vi "GetErrors3.vi"(0 "XRef":T6, 1 "Generate Strings?":T1, 2 "State In":T5) -> (14 "Errors":T2, 15 "Errors Present?":T1)   [LabVIEW 2018, in "OpenG Remove Duplicates from 1 D Array.xnode"]
doc: "This ability VI is used to tell LabVIEW about errors involving your XNode instance. The Errors array is a cluster of errors that will show up as block diagram errors in LabVIEW's error window. The cluster is made up of the errors in the list, the long descriptions of the errors that show up in LabVIEW's error window's details box, and a help file and topic within that file that links this error to the specified help file via the Help button. The help file is the name of the file (*.chm), not the full path and needs to be part of LabVIEW. You only need to populate the array when Generate Strings? is true. You always need to correctly set the Errors Present? indicator. If you are generating strings, then Errors Present? should be true if and only if Errors is not empty. If errors are present, the VI containing the XNode will be broken.\n \n Remeber to localize your errors.\n\nDefault behavior: Generate generic error messages if the code you script is invalid, or a required terminal is unwired.\n\nThis ability does not provide UI and OS messages are not handled."
uses:
  OpenG Remove Duplicates from 1 D Array.xnode
  <vilib>/XNodeSupport/XNodeXNodeRef.ctl
  <vilib>/XNodeSupport/XNodeBool.ctl
  State.ctl
  <vilib>/XNodeSupport/XNodeError3Array.ctl
  <vilib>/XNodeSupport/XNodeError3.ctl
  <vilib>/XNodeSupport/XNodeString.ctl
  <vilib>/XNodeSupport/NI_XNodeSupport.lvlib
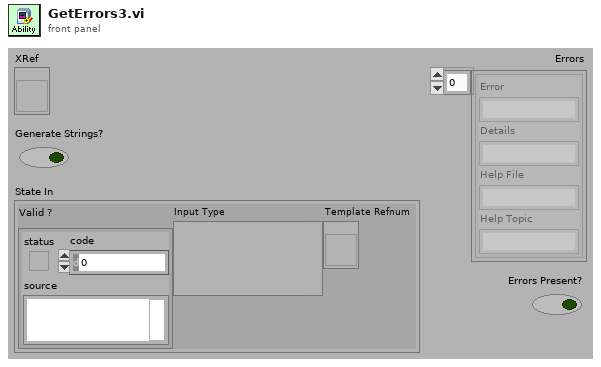
[diagram p1: front panel]
types:
  T1 = typedef "NI_XNodeSupport.lvlib/XNodeBool.ctl" = bool
  T2 = typedef "NI_XNodeSupport.lvlib/XNodeError3Array.ctl" = T3[]
  T3 = typedef "NI_XNodeSupport.lvlib/XNodeError3.ctl" = cluster{"Error":T4, "Details":T4, "Help File":T4, "Help Topic":T4}
  T4 = typedef "NI_XNodeSupport.lvlib/XNodeString.ctl" = string
  T5 = typedef "OpenG Remove Duplicates from 1 D Array.xnode/State.ctl" = cluster{"Valid ?":errorcluster, "Input Type":variant, "Template Refnum":refnum<vi>}
  T6 = typedef "NI_XNodeSupport.lvlib/XNodeXNodeRef.ctl" = refnum<vi>
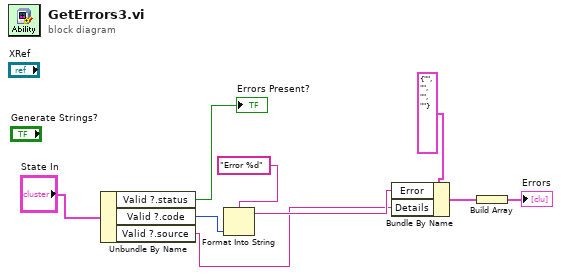
[diagram p0: block diagram]
diagram:
  n1 = Unbundle By Name("State In") -> ("Valid ?.status"=→"Errors Present?":bool, "Valid ?.code"=w8:i32, "Valid ?.source"=w6:string)
  n2 = Format Into String(format string="Error %d", w8) -> (resulting string=w7:string)  [unwired: 2 in, 1 out]
  n3 = Bundle By Name(cluster=T3 {"Error"="", "Details"="", "Help File"="", "Help Topic"=""} ("Error 3"), "Error"=w7, "Details"=w6) -> (w3:T3)
  n4 = Build Array(w3) -> (→"Errors":T3[])
